vi "Get gRPC Device Server Location.vi"(8 "error in":errorcluster, 10 "session name":string, 11 "instrument in":refnum<class "ISession Factory.lvclass">) -> (0 "error out":errorcluster, 2 "remote connection options":T1, 3 "instrument out":refnum<class "ISession Factory.lvclass">)   [LabVIEW 2020, in "MeasurementLink Session Management.lvlib" / "Session Reservation.lvclass"]
uses:
  Session Reservation.lvclass
  Session Reservation.lvclass/Session Reservation.ctl
  MeasurementLink gRPC Utilities/MeasurementLink gRPC Utilities.lvlib
  MeasurementLink gRPC Utilities/TypeDefs/Service Location FGV Action.ctl
  MeasurementLink Discovery Client/RPC Messages/ni_measurementlink_discovery_v1_ResolveServiceRequest.ctl
  MeasurementLink Discovery Client/MeasurementLink Discovery Client.lvlib
  MeasurementLink Instrument/IInstrument/Remote Connection Options.ctl
  MeasurementLink Instrument/IInstrument/ISession Factory.lvclass
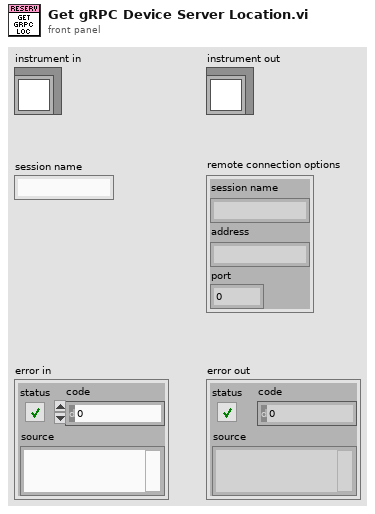
[diagram p1: front panel]
types:
  T1 = typedef "MeasurementLink Instrument.lvlib/ISession Factory.lvclass/Remote Connection Options.ctl" = cluster{"session name":string, "address":string, "port":u32}
  T2 = typedef "MeasurementLink Discovery Client.lvlib/ni_measurementlink_discovery_v1_ResolveServiceRequest.ctl" = cluster{"provided_interface":string, "service_class":string}
  T3 = typedef "MeasurementLink gRPC Utilities.lvlib/Service Location FGV Action.ctl" = enum16{"Get Service Location", "Clear Cache"}
  T4 = typedef "MeasurementLink Discovery Client.lvlib/ni_measurementlink_discovery_v1_ServiceLocation.ctl" = cluster{"location":string, "insecure_port":string, "ssl_authenticated_port":string}
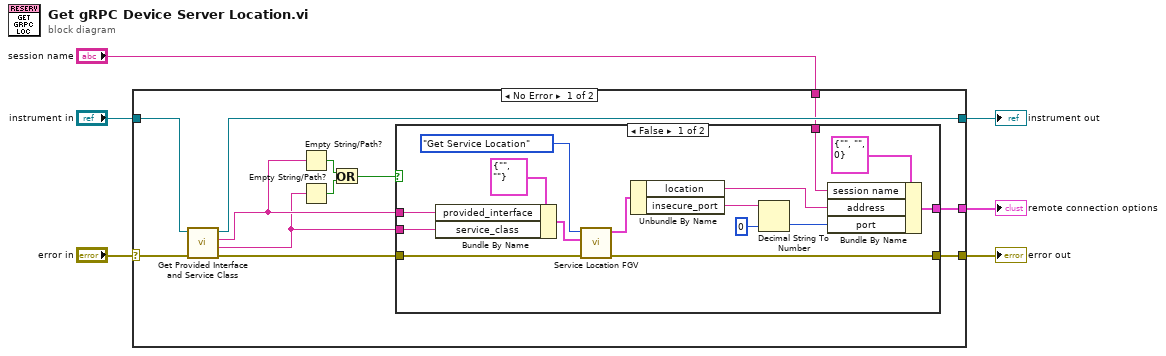
[diagram p0: block diagram]
diagram:
  n1 = case shown="No Error" "error in" {
    selector: "error in" -> [w14 w36]
    tunnel: [w18 w36] -> w6
    tunnel: [w17 w35] -> w5
    tunnel: "instrument in" -> [w15 w35]
    tunnel: [w13 _] -> w2
    tunnel: "session name" -> [w12 _]
    frame No Error {
      n2 = call-dynamic "Get Provided Interface and Service Class.vi"("error in (no error)"=w14, "instrument in"=w15) -> ("error out"=w16:errorcluster, "service class"=w7:string, "provided interface"=w11:string, "instrument out"=w17:refnum<class "ISession Factory.lvclass">)  [unwired: 6 in]
      n3 = Empty String/Path?(string/path=w11) -> (empty?=w10:bool)
      n4 = Empty String/Path?(string/path=w7) -> (empty?=w9:bool)
      n5 = Or(x=w10, y=w9) -> (x .or. y?=w8:bool)
      n6 = case shown="False" w8 {
        tunnel: [w30 w34] -> w18
        tunnel: w7 -> [w29 _]
        tunnel: w11 -> [w28 _]
        tunnel: w16 -> [w24 w34]
        tunnel: [w20 _] -> w13
        tunnel: w12 -> [w19 _]
        frame False {
          n7 = Bundle By Name(cluster=T2 {"provided_interface"="", "service_class"=""} ("Resolve Service Request"), "provided_interface"=w28, "service_class"=w29) -> (w25:T2)
          n8 = call "Service Location FGV.vi"("error in"=w24, "Resolve Service Request"=w25, "Action"=Service_Location_FGV_Action."Get Service Location") -> ("error out"=w30:errorcluster, "Service Location"=w32:T4)  [unwired: 7 in]
          n9 = Unbundle By Name(w32) -> ("location"=w22:string, "insecure_port"=w31:string)
          n10 = Decimal String To Number(string=w31, default (0L)=u32 0 ("default (0 I32)")) -> (number=w21:u32)  [unwired: 1 in, 1 out]
          n11 = Bundle By Name(cluster=T1 {"session name"="", "address"="", "port"=0} ("remote connection options"), "session name"=w19, "address"=w22, "port"=w21) -> (w20:T1)
        }
        frame True {
        }
      }
    }
    frame Error {
    }
  }
  "error out" <- w6
  "instrument out" <- w5
  "remote connection options" <- w2
